vi "Recieve Result.vi"(8 "error in (no error)":errorcluster, 10 "Mag Lab Result.lvclass":refnum<class "Mag Lab Result.lvclass">, 11 "Cap Bank Server in":refnum<class "Cap Bank Server.lvclass">) -> (0 "error out":errorcluster, 3 "Cap Bank Server out":refnum<class "Cap Bank Server.lvclass">)   [LabVIEW 2012]
uses:
  Mag Lab Result/Mag Lab Result.lvclass
  User Cap Bank/Labview/Library/Shot data.ctl
  Cap Bank Server.lvclass
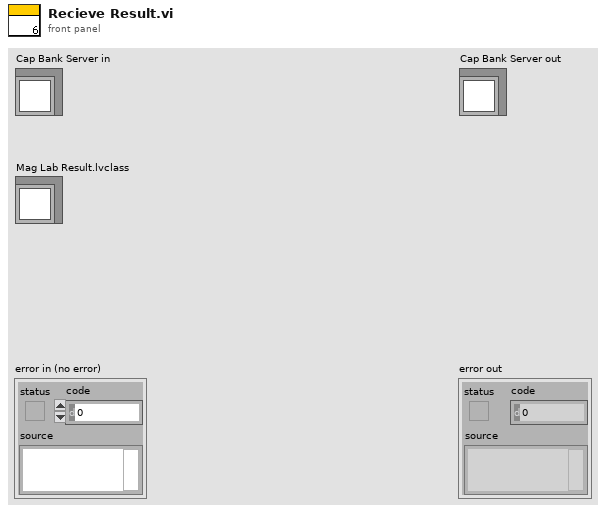
[diagram p1: front panel]
types:
  T1 = typedef "Shot data.ctl" = cluster{"Shot number":i32, "Time":timestamp, "Magnet ID":string, "User":string, "Cell number":i32, "Requested field":dbl, "Field direction":string, "Number of bank frames":i32, "Crowbar resistance, mOhm":dbl, "Magnet resistance, mOhm":dbl, "Charger voltage, kV":dbl, "Frame voltage, kV":dbl}
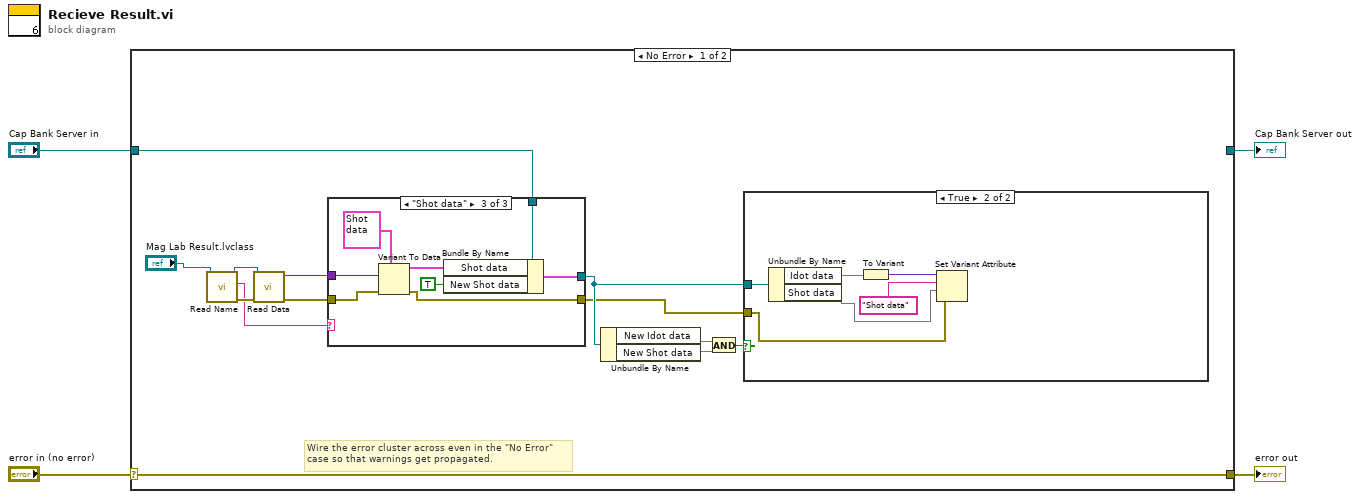
[diagram p0: block diagram]
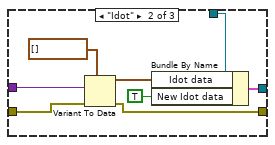
[diagram p4: hidden frame]
diagram:
  n1 = case shown="No Error" "error in (no error)" {
    selector: "error in (no error)" -> [w17 w43]
    tunnel: [w17 w43] -> w3
    tunnel: [_ w42] -> w1
    tunnel: "Cap Bank Server in" -> [w10 w42]
    frame No Error {
      # "Wire the error cluster across even in the \"No Error\"\ncase so that warnings get propagated."
      n2 = call "Read Name.vi"("Mag Lab Result in"="Mag Lab Result.lvclass") -> ("error out"=w16:errorcluster, "Name"=w12:string, "Mag Lab Result out"=w13:refnum<class "Mag Lab Result.lvclass">)  [unwired: 8 in]
      n3 = call "Read Data.vi"("error in (no error)"=w16, "Mag Lab Result in"=w13) -> ("error out"=w15:errorcluster, "Data"=w14:variant)  [unwired: 7 in, 1 out]
      n4 = case shown="\"Shot data\"" w12 {
        tunnel: w14 -> [_ w32 w41]
        tunnel: w15 -> [w24 w31 w40]
        tunnel: w10 -> [w25 w30 w39]
        tunnel: [w25 w27 w36] -> w6
        tunnel: [w24 w26 w34] -> w5
        frame "", Default {
        }
        frame "Idot" {
          n5 = Variant To Data(error in=w31, type=waveform(dbl)[] [] ("data"), Variant=w32) -> (data=w29:waveform(dbl)[], error out=w26:errorcluster)
          n6 = Bundle By Name(cluster=w30, "Idot data"=w29, "New Idot data"=TRUE) -> (w27:cluster{})
        }
        frame "Shot data" {
          n7 = Variant To Data(error in=w40, type=T1 {"Shot number"=0, "Time"=timestamp(0 s since 1904-01-01), "Magnet ID"="", "User"="", "Cell number"=0, "Requested field"=0.0, "Field direction"="", "Number of bank frames"=0, "Crowbar resistance, mOhm"=0.0, "Magnet resistance, mOhm"=0.0, "Charger voltage, kV"=0.0, "Frame voltage, kV"=0.0} ("Shot data"), Variant=w41) -> (data=w38:T1, error out=w34:errorcluster)
          n8 = Bundle By Name(cluster=w39, "Shot data"=w38, "New Shot data"=TRUE ("New Idot data")) -> (w36:cluster{})
        }
      }
      n9 = Unbundle By Name(w6) -> ("New Idot data"=w9, "New Shot data"=w8)
      n10 = And(x=w9, y=w8) -> (x .and. y?=w7:bool)
      n11 = case shown="True" w7 {
        tunnel: w6 -> [_ w23]
        tunnel: w5 -> [_ w18]
        frame False {
        }
        frame True {
          n12 = Unbundle By Name(w23) -> ("Idot data"=w22, "Shot data"=w19)
          n13 = To Variant(anything=w22) -> (Variant=w21:variant)
          n14 = Set Variant Attribute(Variant=w21, name="Shot data", value=w19, error in=w18) -> ()  [unwired: 3 out]
        }
      }
    }
    frame Error {
    }
  }
  "error out" <- w3
  "Cap Bank Server out" <- w1
